vi "PrefDialog.vi"(8 "error in (no error)":errorcluster, 11 "MyPluginsBase in":refnum<class "NHRGridSim.lvclass">) -> (0 "error out":errorcluster, 1 "Save As":bool, 2 "Changed":bool, 3 "MyPluginsBase out":refnum<class "NHRGridSim.lvclass">)   [LabVIEW 2018, in "AcPwrPlugins.lvlib" / "NHRGridSim.lvclass"]
doc: "This VI opens up the modal preference dialog window and allows a user to configure the properties with new values, or keep the existing values from the last time the function was called. The user can also save the new values to a new file name and new type name using the save as button."
uses:
  NHRGridSim.lvclass
  C:/Program Files (x86)/National Instruments/LabVIEW 2018/user.lib/NIST/BaseClasses/BasePlugin_class/BasePlugin.lvclass
  C:/Users/ico/Documents/Projects/NistPluggableModules/AcPwr/AcPwrPlugins/AcPwrBaseClass/AcPwrBase.lvclass
  TypeDefs/Device(s)Settings.ctl
  TypeDefs/Modules.ctl
  Measurements.ctl
  TypeDefs/MeasurementType.ctl
  <userlib>/NIST/BaseClasses/BasePlugin_class/BasePlugin.lvclass/BasePlugin.ctl
  AcPwrBaseClass/AcPwrBase.lvclass/AcPwrBase.ctl
  <userlib>/NIST/BaseClasses/BasePlugin_class/Accessors/Read PluginIniFilePath.vi
  AcPwrBaseClass/Accessors/Read BaseConfig.vi
  AcPwrBaseClass/Accessors/Read BaseMeasurements.vi
  <userlib>/NIST/BaseClasses/BasePlugin_class/Accessors/Write PluginIniFilePath.vi
  <vilib>/Utility/config.llb/NI_LVConfig.lvlib
  AcPwrBaseClass/AcPwrBase.lvclass
panel:
  in  "Measurements":T1 {"Phase" items=["All", "A Phase", "B Phase", "C Phase"]}
  in  "Device(s)Settings":T3 {"Modules"."Phase (0: All)" items=["All", "A Phase", "B Phase", "C Phase"]; "Modules"."Mode" items=["One 3-Phase AC", "One AC", "One DC", "Three AC", "Three DC", "One 2-Phase AC and One AC", "One 2-Phase AC and One DC", "Two AC", "One AC and One DC", "Two AC and One DC", "One AC and Two DC", "One DC and One AC", "Two DC"]}
  in  "btnSaveAs":bool
  in  "Measurement RefreshTime (ms)":u32
  in  "btnSave":bool
  in  "btnCancel":bool
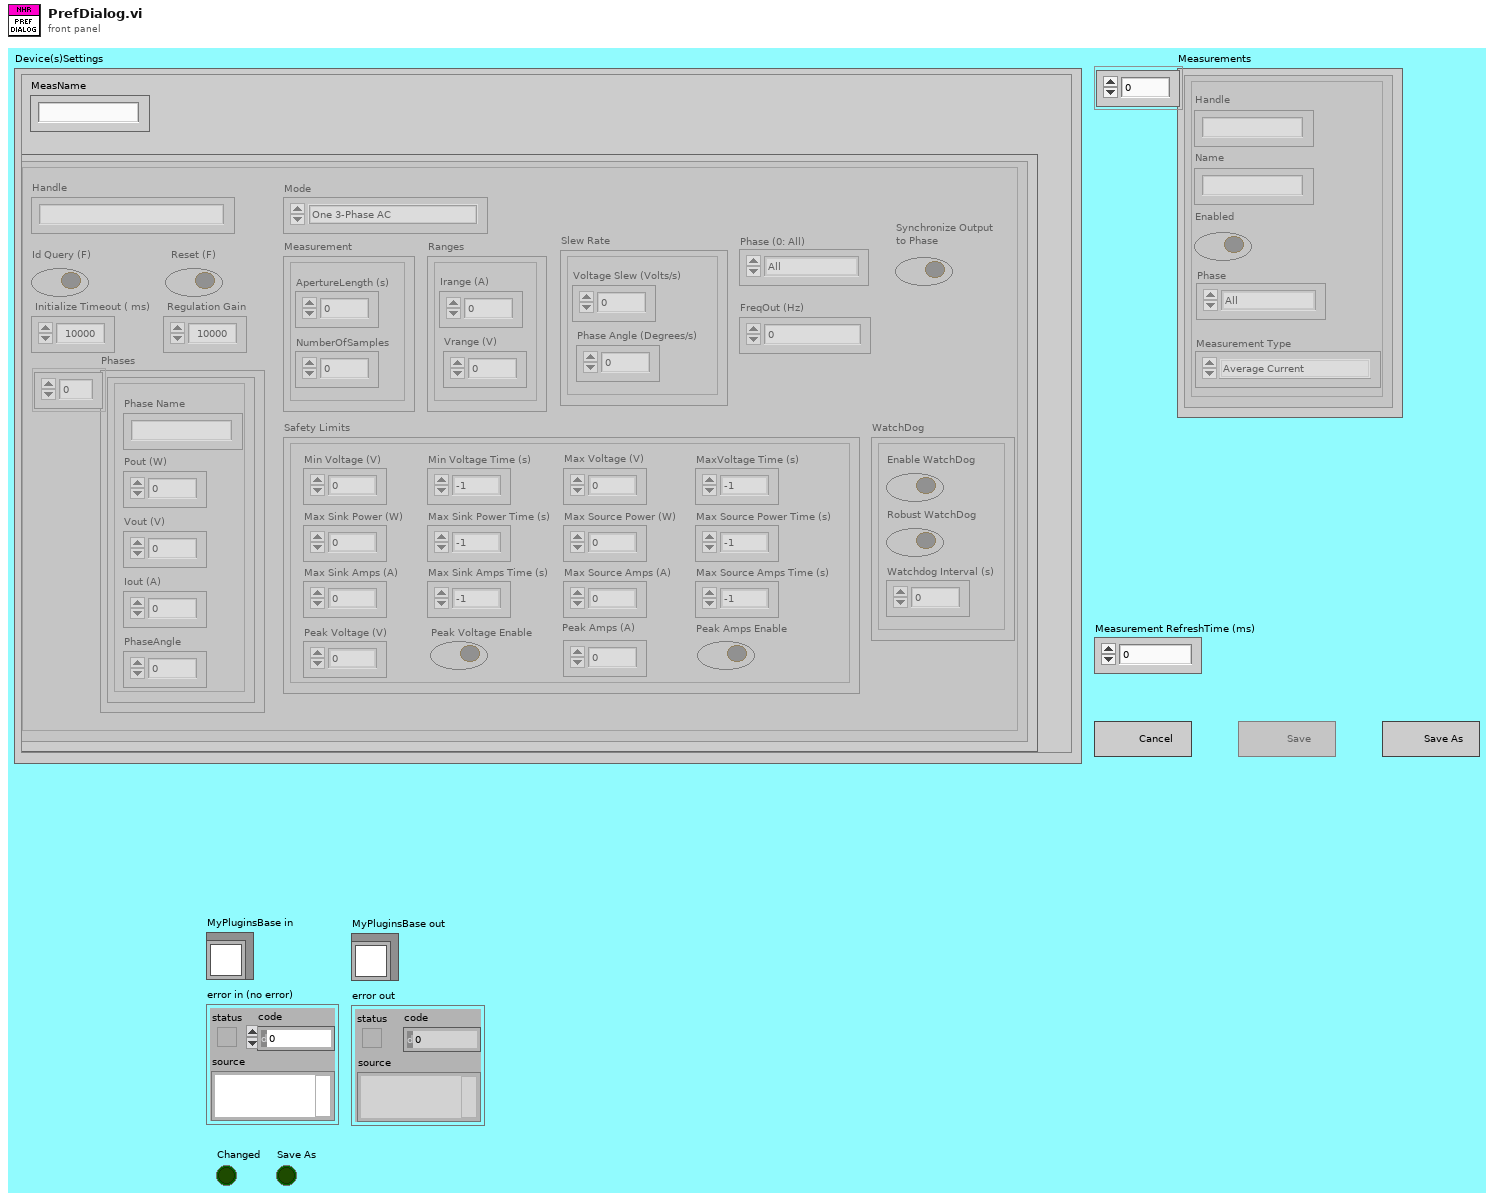
[diagram p1: front panel]
types:
  T1 = typedef "AcPwrPlugins.lvlib/NHRGridSim.lvclass/Measurements.ctl" = cluster{"Handle":string, "Name":string, "Enabled ":bool, "Measurement Value":dbl, "Phase ":i32, "Measurement Type ":T2}[]
  T2 = typedef "AcPwrPlugins.lvlib/NHRGridSim.lvclass/MeasurementType.ctl" = enum16{"Average Current", "Average Voltage"}
  T3 = typedef "AcPwrPlugins.lvlib/NHRGridSim.lvclass/Device(s)Settings.ctl" = cluster{"MeasName":string, "Modules":T4}
  T4 = typedef "AcPwrPlugins.lvlib/NHRGridSim.lvclass/Modules.ctl" = cluster{"Measurement":cluster{"ApertureLength (s)":dbl, "NumberOfSamples":u32}, "Ranges":cluster{"Irange (A)":dbl, "Vrange (V)":dbl}, "Mode":u8, "Handle":string, "FreqOut (Hz)":dbl, "Connected":bool, "btnIdQuery":bool, "btnReset":bool, "Initialize Timeout ( ms)":u32, "Phase (0: All)":i32, "WatchDog":cluster{"Enable WatchDog":bool, "Robust WatchDog":bool, "Watchdog Interval (s)":dbl}, "Safety Limits":cluster{"Min Voltage (V)":dbl, "Min Voltage Time (s)":dbl, "Max Voltage (V)":dbl, "MaxVoltage Time (s)":dbl, "Max Source Amps (A)":dbl, "Max Source Amps Time (s)":dbl, "Max Sink Amps (A)":dbl, "Max Sink Amps Time (s)":dbl, "Max Source Power (W)":dbl, "Max Source Power Time (s)":dbl, "Max Sink Power (W)":dbl, "Max Sink Power Time (s)":dbl, "Peak Voltage (V)":dbl, "Peak Voltage Enable":bool, "Peak Amps (A)":dbl, "Peak Amps Enable":bool}, "Phases":cluster{"Pout (W)":dbl, "Iout (A)":dbl, "PhaseAngle":dbl, "Vout (V)":dbl, "Phase Name":string}[], "Regulation Gain":dbl, "ChangeOntheFly":bool, "Synchronize Output \nto Phase":bool, "Slew Rate":cluster{"Voltage Slew (Volts/s)":dbl, "Phase Angle (Degrees/s)":dbl}}[]
  T5 = enum32{"Invalid", "Standard", "Closed", "Hidden", "Minimized", "Maximized"}
  T6 = enum32{"Invalid", "Default", "Floating", "Floating/Auto-Hide", "Modal"}
  T7 = enum8{"Enabled", "Disabled", "Disabled and Grayed Out"}
  T8 = typedef "AcPwrPlugins.lvlib/AcPwrBase.lvclass/BaseConfig.ctl" = cluster{"Frequency":dbl, "FrequencyRange":dbl[], "Phases":T9[], "Name":string, "PluginConfigVariant":variant, "PluginMeasVariant":variant}
  T9 = typedef "AcPwrPlugins.lvlib/AcPwrBase.lvclass/Phase.ctl" = cluster{"Name":string, "Enabled":bool, "VoltageLevel":dbl, "Handle":string, "VoltageRange":dbl[], "Connected":bool, "CurrentLimit":dbl, "Waveform":string}
  T10 = typedef "AcPwrPlugins.lvlib/AcPwrBase.lvclass/BaseMeasurements.ctl" = cluster{"Handle":string, "Name":string, "Enabled":bool, "Measurement Value":dbl, "btnMeasFetch":bool, "Chroma Hold Peak Current Measurement":bool, "Chroma Measurement Type":T11, "Chroma Protection Status String":string, "NHRDC Fetch Method":i32, "NHRDC Fetch Time (s)":sgl, "NHRDC Measurement Type":i32, "NHRGridSim Measurement Type ":enum16{"Average Current", "Max Current", "Min Current", "Average Voltage", "Max Voltage", "Min Voltage", "Average True Power", "Max True Power", "Min True Power", "Average Apparent Power", "Max Apparent Power", "Min Apparent Power", "Power Factor", "Crest Factor"}, "NHRGridSim Phase ":i32, "PPS Measurement Type ":enum16{"Voltage RMS L-N", "Voltage RMS L-L", "Frequency", "Current RMS", "Current Peak", "Crest Factor", "Power Factor", "Power VA", "Real Power"}, "PPS Channel Name":enum16{"A", "B", "C"}}[]
  T11 = typedef "AcPwrPlugins.lvlib/ChromaAcLoad.lvclass/MeasurementType.ctl" = enum16{"Voltage (Vrms or V)", "Current (Arms or A)", "Power (W)", "Peak Voltage (V)", "Peak Current (A)", "Peak Power (W)", "Frequency (Hz)", "Resistance (Ohms)", "Voltage Overshoot (V)", "Positive Peak Current (A)", "Voltage Undershoot (V)", "Negative Peak Current (A)", "Apparent Power (VA)", "Reacitive Power (VAR)", "Voltage THD", "Power Factor", "Current's Crest Factor"}
  T12 = cluster{"Measurement":cluster{"ApertureLength (s)":dbl, "NumberOfSamples":u32}, "Ranges":cluster{"Irange (A)":dbl, "Vrange (V)":dbl}, "Mode":u8, "Handle":string, "FreqOut (Hz)":dbl, "Connected":bool, "btnIdQuery":bool, "btnReset":bool, "Initialize Timeout ( ms)":u32, "Phase (0: All)":i32, "WatchDog":cluster{"Enable WatchDog":bool, "Robust WatchDog":bool, "Watchdog Interval (s)":dbl}, "Safety Limits":cluster{"Min Voltage (V)":dbl, "Min Voltage Time (s)":dbl, "Max Voltage (V)":dbl, "MaxVoltage Time (s)":dbl, "Max Source Amps (A)":dbl, "Max Source Amps Time (s)":dbl, "Max Sink Amps (A)":dbl, "Max Sink Amps Time (s)":dbl, "Max Source Power (W)":dbl, "Max Source Power Time (s)":dbl, "Max Sink Power (W)":dbl, "Max Sink Power Time (s)":dbl, "Peak Voltage (V)":dbl, "Peak Voltage Enable":bool, "Peak Amps (A)":dbl, "Peak Amps Enable":bool}, "Phases":cluster{"Pout (W)":dbl, "Iout (A)":dbl, "PhaseAngle":dbl, "Vout (V)":dbl, "Phase Name":string}[], "Regulation Gain":dbl, "ChangeOntheFly":bool, "Synchronize Output \nto Phase":bool, "Slew Rate":cluster{"Voltage Slew (Volts/s)":dbl, "Phase Angle (Degrees/s)":dbl}}
  T13 = typedef "NI_LVConfig.lvlib/Config Data RefNum.ctl" = refnum<k1>
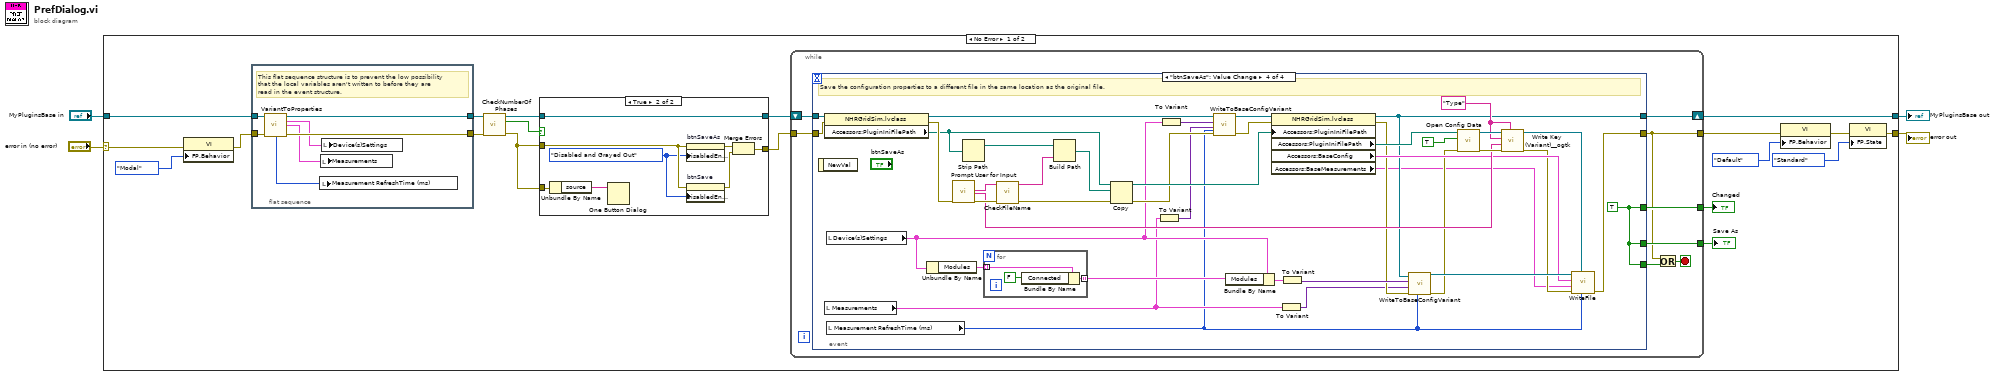
[diagram p0: block diagram]
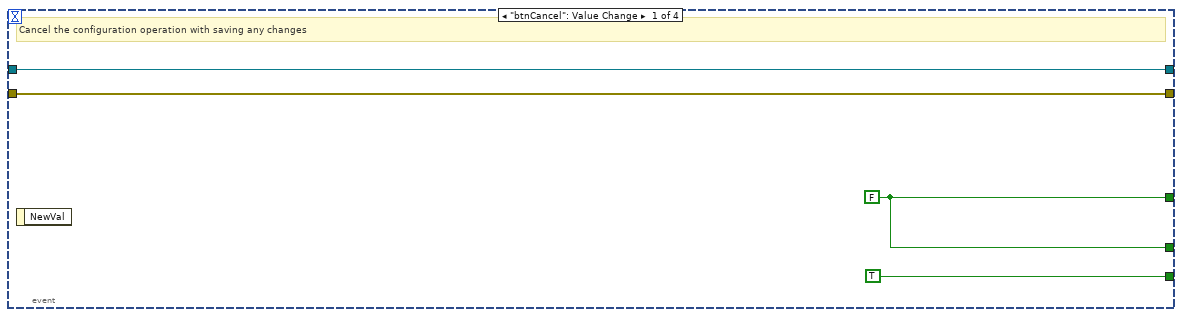
[diagram p2: hidden frame]
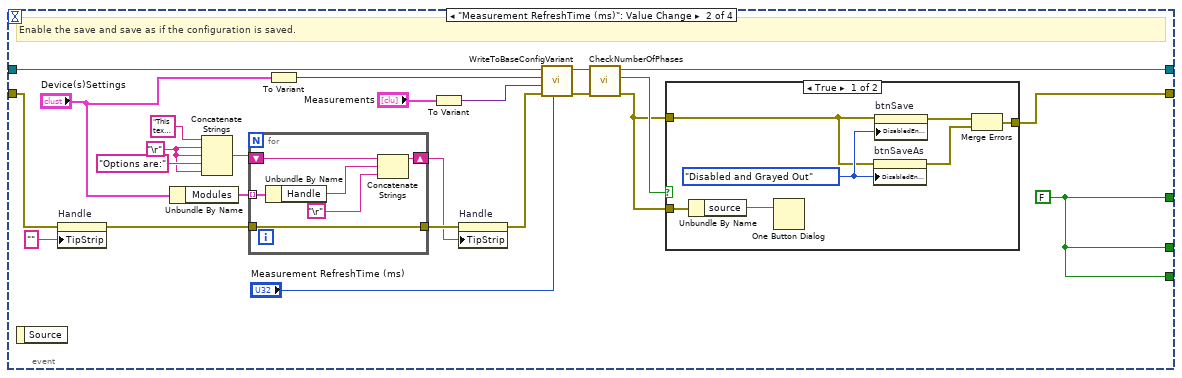
[diagram p3: hidden frame]
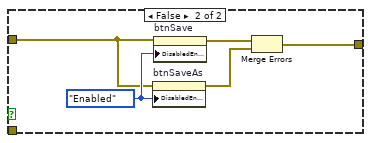
[diagram p4: hidden frame]
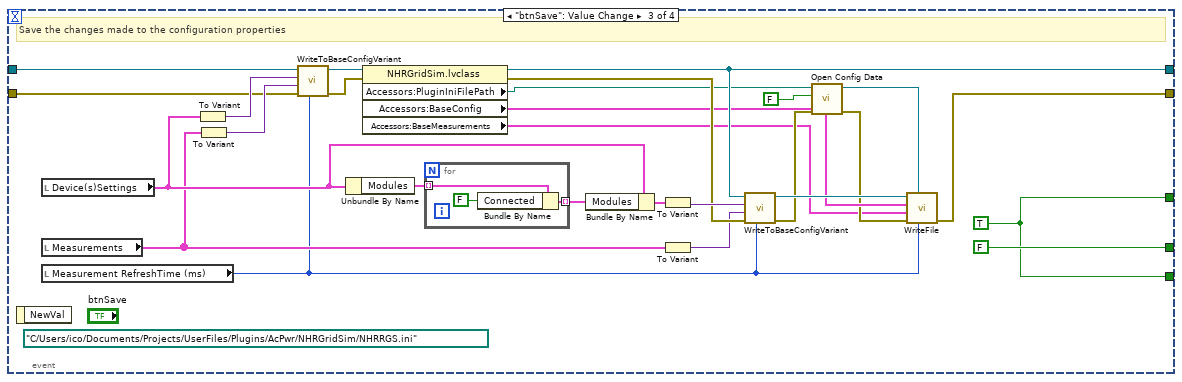
[diagram p5: hidden frame]
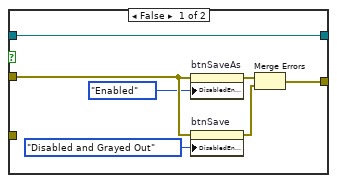
[diagram p6: hidden frame]
diagram:
  n1 = case shown="No Error" "error in (no error)" {
    selector: "error in (no error)" -> [w21 w175]
    tunnel: "MyPluginsBase in" -> [w16 w174]
    tunnel: [w14 w174] -> w2
    tunnel: [w12 w175] -> w1
    frame No Error {
      n2 = property class="VI"(error in=w21, "FP.Behavior"=T6."Modal" ("Front Panel Window:Behavior")) -> (error out=w17:errorcluster)  [unwired: 1 in, 1 out]
      n3 = flat-sequence {
        tunnel: w16 -> [w30]
        tunnel: [w29] -> w9
        tunnel: [w27] -> w10
        tunnel: w17 -> [w28]
        frame #0 {
          # "This flat sequence structure is to prevent the low possibility that the local variables aren't written to before they are read in the event structure."
          n4 = call "VariantToProperties.vi"("NHRGridSim in"=w30, "error in (no error)"=w28) -> ("NHRGridSim out"=w29:refnum<class "NHRGridSim.lvclass">, "Device(s)Settings"=w26:T3, "Measurements"=w24:T1, "Measurement Refresh Time (ms)"=w25:u32, "error out"=w27:errorcluster)  [unwired: 7 in, 2 out]
          n5 = local write "Measurement RefreshTime (ms)"(w25) -> ()
          n6 = local write "Measurements"(w24) -> ()
          n7 = local write "Device(s)Settings"(w26) -> ()
        }
      }
      n8 = call "CheckNumberOfPhases.vi"("error in (no error)"=w10, "NHRGridSim in"=w9) -> ("error out"=w7:errorcluster, "Boolean"=w8:bool, "NHRGridSim out"=w6:refnum<class "NHRGridSim.lvclass">)  [unwired: 6 in, 1 out]
      n9 = case shown="True" w8 {
        tunnel: w7 -> [w164 w172]
        tunnel: [w163 w171] -> w15
        tunnel: w7 -> [_ w168]
        tunnel: w6 -> [w159 w166]
        tunnel: [w159 w166] -> w5
        frame False {
          # "Check if the number of Phases=Loads. If no disables the ability\nto save as."
          n10 = property on="btnSaveAs" class="Bool"(error in=w164, "DisabledEnum"=T7."Enabled" ("Disabled")) -> (error out=w165:errorcluster)  [unwired: 1 in, 1 out]
          n11 = property on="btnSave" class="Bool"(error in=w164, "DisabledEnum"=T7."Disabled and Grayed Out" ("Disabled")) -> (error out=w162:errorcluster)  [unwired: 1 in, 1 out]
          n12 = Merge Errors(w165, w162) -> (w163:errorcluster)
        }
        frame True {
          w169 = T7."Disabled and Grayed Out" ("Disabled")
          # "Check if the number of Phases=Loads. If no disables the ability\nto save as."
          n13 = Unbundle By Name(w168) -> ("source"=w167:string)
          n14 = One Button Dialog(message=w167) -> ()  [unwired: 1 in, 1 out]
          n15 = property on="btnSaveAs" class="Bool"(error in=w172, "DisabledEnum"=w169) -> (error out=w173:errorcluster)  [unwired: 1 in, 1 out]
          n16 = property on="btnSave" class="Bool"(error in=w172, "DisabledEnum"=w169) -> (error out=w170:errorcluster)  [unwired: 1 in, 1 out]
          n17 = Merge Errors(w173, w170) -> (w171:errorcluster)
        }
      }
      n18 = while {
        shift-right: [w36] -> w14
        shift-left: w5 -> [w37]
        tunnel: [w38] -> w22
        tunnel: [w34] -> w13
        tunnel: w15 -> [w35]
        tunnel: [w31] -> w11
        stop <- w33 stop-if-true
        n19 = event shown="[3] \"btnSaveAs\": Value Change" {
          selector: _ -> [_ _ _ _]
          dyn-events: _ -> [_ _ _ _]
          timeout: _ -> [_ _ _ _]
          tunnel: [w39 w65 w109 w150] -> w38
          tunnel: [TRUE w65 w109 w150] -> w32
          tunnel: w37 -> [w41 w57 w90 w144]
          tunnel: [w41 w60 w104 w128] -> w36
          tunnel: [w40 w66 w106 w130] -> w31
          tunnel: w35 -> [w40 w50 w87 w143]
          tunnel: [w39 w65 FALSE w150] -> w34
          event "btnCancel": Value Change {
            w39 = FALSE
            # "Cancel the configuration operation with saving any changes"
            n20 = event-data() -> ()  [unwired: 1 in, 1 out]
          }
          event "Measurement RefreshTime (ms)": Value Change {
            w62 = "\r"
            w65 = FALSE
            # "Enable the save and save as if the configuration is saved."
            n21 = event-data() -> ()  [unwired: 1 in, 1 out]
            n22 = property on="Handle" class="Str"(error in=w50, "TipStrip"="" ("Tip Strip")) -> (error out=w49:errorcluster)  [unwired: 1 in, 1 out]
            n23 = Unbundle By Name("Device(s)Settings") -> ("Modules"=w53:T4)
            n24 = Concatenate Strings("This text in this handle of the instrument and entered in the  \nhandle control in the Phases array EXACTLY, lest the attempt \nto interact with the instrument will fail.", w62, w62, "Options are:" ("Handle"), w62) -> (w61:string)
            n25 = for {
              shift-right: [w72] -> w46
              shift-left: w61 -> [w71]
              tunnel: w53 -> [w70] mode=indexing
              tunnel: w49 -> [w67]
              tunnel: [w67] -> w47
              n26 = Unbundle By Name(w70) -> ("Handle"=w69:string)
              n27 = Concatenate Strings(w71, w69, "\r") -> (w72:string)
            }
            n28 = To Variant(anything="Device(s)Settings") -> (Variant=w58:variant)
            n29 = To Variant(anything="Measurements") -> (Variant=w43:variant)
            n30 = property on="Handle" class="Str"(error in=w47, "TipStrip"=w46) -> (error out=w48:errorcluster)  [unwired: 1 in, 1 out]
            n31 = call "WriteToBaseConfigVariant.vi"("Measurement RefreshTime (ms)"="Measurement RefreshTime (ms)", "error in (no error)"=w48, "Meas"=w43, "Config"=w58, "NHRGridSim in"=w57) -> ("error out"=w55:errorcluster, "NHRGridSim out"=w56:refnum<class "NHRGridSim.lvclass">)  [unwired: 5 in]
            n32 = call "CheckNumberOfPhases.vi"("error in (no error)"=w55, "NHRGridSim in"=w56) -> ("error out"=w54:errorcluster, "Boolean"=w59:bool, "NHRGridSim out"=w60:refnum<class "NHRGridSim.lvclass">)  [unwired: 6 in, 1 out]
            n33 = case shown="True" w59 {
              tunnel: w54 -> [w76 w81]
              tunnel: [w75 w80] -> w66
              tunnel: w54 -> [w73 _]
              frame True {
                w77 = T7."Disabled and Grayed Out" ("Disabled")
                n34 = Unbundle By Name(w73) -> ("source"=w74:string)
                n35 = One Button Dialog(message=w74) -> ()  [unwired: 1 in, 1 out]
                n36 = property on="btnSaveAs" class="Bool"(error in=w76, "DisabledEnum"=w77) -> (error out=w79:errorcluster)  [unwired: 1 in, 1 out]
                n37 = property on="btnSave" class="Bool"(error in=w76, "DisabledEnum"=w77) -> (error out=w78:errorcluster)  [unwired: 1 in, 1 out]
                n38 = Merge Errors(w78, w79) -> (w75:errorcluster)
              }
              frame False {
                w82 = T7."Enabled" ("Disabled")
                n39 = property on="btnSaveAs" class="Bool"(error in=w81, "DisabledEnum"=w82) -> (error out=w84:errorcluster)  [unwired: 1 in, 1 out]
                n40 = property on="btnSave" class="Bool"(error in=w81, "DisabledEnum"=w82) -> (error out=w83:errorcluster)  [unwired: 1 in, 1 out]
                n41 = Merge Errors(w83, w84) -> (w80:errorcluster)
              }
            }
          }
          event "btnSave": Value Change {
            (unwired) path "C:/Users/ico/Documents/Projects/UserFiles/Plugins/AcPwr/NHRGridSim/NHRRGS.ini" ("Accessors:PluginIniFilePath")
            w109 = TRUE ("StartMeas")
            # "Save the changes made to the configuration properties"
            n42 = event-data() -> ()  [unwired: 1 in, 1 out]
            n43 = local read "Device(s)Settings"() -> (w89:T3)
            n44 = local read "Measurements"() -> (w88:T1)
            n45 = local read "Measurement RefreshTime (ms)"() -> (w86:u32)
            n46 = To Variant(anything=w89) -> (Variant=w94:variant)
            n47 = To Variant(anything=w88) -> (Variant=w93:variant)
            n48 = call "WriteToBaseConfigVariant.vi"("Measurement RefreshTime (ms)"=w86, "error in (no error)"=w87, "Meas"=w93, "Config"=w94, "NHRGridSim in"=w90) -> ("error out"=w91:errorcluster, "NHRGridSim out"=w92:refnum<class "NHRGridSim.lvclass">)  [unwired: 5 in]
            n49 = Unbundle By Name(w89) -> ("Modules"=w107:T4)
            n50 = property class="NHRGridSim.lvclass"(reference=w92, error in=w91) -> (reference out=w104:refnum<class "NHRGridSim.lvclass">, error out=w101:errorcluster, "Accessors:PluginIniFilePath"=w85:path, "Accessors:BaseConfig"=w100:T8, "Accessors:BaseMeasurements"=w97:T10)
            n51 = for {
              tunnel: w107 -> [w114] mode=indexing
              tunnel: [w113] -> w108 mode=indexing
              n52 = Bundle By Name(cluster=w114, "Connected"=FALSE) -> (w113:T12)
            }
            n53 = Bundle By Name(cluster=w89, "Modules"=w108) -> (w96:T3)
            n54 = To Variant(anything=w96) -> (Variant=w105:variant)
            n55 = To Variant(anything=w88) -> (Variant=w95:variant)
            n56 = call "WriteToBaseConfigVariant.vi"("Measurement RefreshTime (ms)"=w86, "error in (no error)"=w101, "Meas"=w95, "Config"=w105, "NHRGridSim in"=w104) -> ("error out"=w102:errorcluster, "NHRGridSim out"=w103:refnum<class "NHRGridSim.lvclass">)  [unwired: 5 in]
            n57 = call <vilib>:"Open Config Data.vi"("error in (no error)"=w102, "create file if necessary (T)"=FALSE, "configuration file path"=w85) -> ("error out"=w98:errorcluster, "refnum"=w99:T13)  [unwired: 6 in, 1 out]
            n58 = call-dynamic "WriteFile.vi"("RefreshTime"=w86, "Refnum in"=w99, "error in (no error)"=w98, "BaseMeasurements"=w97, "BaseConfiguration"=w100, "NHRGridSim in"=w103) -> ("error out"=w106:errorcluster)  [unwired: 4 in, 1 out]
          }
          event "btnSaveAs": Value Change {
            w145 = "Type" ("section (optional)")
            w150 = TRUE
            # "Save the configuration properties to a different file in the same location as the original file."
            n59 = event-data() -> ()  [unwired: 1 in, 1 out]
            n60 = property class="NHRGridSim.lvclass"(reference=w144, error in=w143) -> (reference out=w120:refnum<class "NHRGridSim.lvclass">, error out=w142:errorcluster, "Accessors:PluginIniFilePath"=w141:path)
            n61 = local read "Measurements"() -> (w117:T1)
            n62 = local read "Device(s)Settings"() -> (w118:T3)
            n63 = local read "Measurement RefreshTime (ms)"() -> (w115:u32)
            n64 = Unbundle By Name(w118) -> ("Modules"=w138:T4)
            n65 = call "Prompt User for Input"("error in (no error)"=w142) -> ("File Name"=w140:string, "PluginType"=w146:string, "error out"=w147:errorcluster)  [unwired: 15 in, 1 out]
            n66 = Strip Path(path=w141) -> (stripped path=w152:path)  [unwired: 1 out]
            n67 = for {
              tunnel: w138 -> [w158] mode=indexing
              tunnel: [w157] -> w139 mode=indexing
              n68 = Bundle By Name(cluster=w158, "Connected"=FALSE) -> (w157:T12)
            }
            n69 = call "CheckFileName.vi"("Error In"=w147, "File Name in"=w140) -> ("Error Out"=w148:errorcluster, "File Name out"=w149:string)  [unwired: 8 in]
            n70 = Build Path(base path=w152, name or relative path=w149) -> (appended path=w151:path)
            n71 = Copy(8:w148, 10:w151, 11:w141) -> (0:w123:errorcluster, 3:w134:path)  [unwired: 2 in, 1 out]
            n72 = To Variant(anything=w117) -> (Variant=w116:variant)
            n73 = To Variant(anything=w118) -> (Variant=w119:variant)
            n74 = call "WriteToBaseConfigVariant.vi"("Measurement RefreshTime (ms)"=w115, "error in (no error)"=w123, "Meas"=w116, "Config"=w119, "NHRGridSim in"=w120) -> ("error out"=w122:errorcluster, "NHRGridSim out"=w121:refnum<class "NHRGridSim.lvclass">)  [unwired: 5 in]
            n75 = Bundle By Name(cluster=w118, "Modules"=w139) -> (w137:T3)
            n76 = property class="NHRGridSim.lvclass"(reference=w121, error in=w122, "Accessors:PluginIniFilePath"=w134) -> (reference out=w128:refnum<class "NHRGridSim.lvclass">, error out=w129:errorcluster, "Accessors:PluginIniFilePath"=w133:path, "Accessors:BaseConfig"=w132:T8, "Accessors:BaseMeasurements"=w125:T10)
            n77 = To Variant(anything=w117) -> (Variant=w124:variant)
            n78 = To Variant(anything=w137) -> (Variant=w136:variant)
            n79 = call "WriteToBaseConfigVariant.vi"("Measurement RefreshTime (ms)"=w115, "error in (no error)"=w129, "Meas"=w124, "Config"=w136, "NHRGridSim in"=w128) -> ("error out"=w127:errorcluster, "NHRGridSim out"=w135:refnum<class "NHRGridSim.lvclass">)  [unwired: 5 in]
            n80 = call <vilib>:"Open Config Data.vi"("error in (no error)"=w127, "create file if necessary (T)"=TRUE, "configuration file path"=w133) -> ("error out"=w154:errorcluster, "refnum"=w153:T13)  [unwired: 6 in, 1 out]
            n81 = call <userlib>:"Write Key (Variant)__ogtk.vi"("section"=w145, "error in (no error)"=w154, "key-value"=w146, "key (optional)"=w145, "refnum"=w153) -> ("error out"=w126:errorcluster, "refnum out"=w131:T13)  [unwired: 5 in]
            n82 = call-dynamic "WriteFile.vi"("RefreshTime"=w115, "Refnum in"=w131, "error in (no error)"=w126, "BaseMeasurements"=w125, "BaseConfiguration"=w132, "NHRGridSim in"=w135) -> ("error out"=w130:errorcluster)  [unwired: 4 in, 1 out]
          }
        }
        n83 = Or(x=w31, y=w32) -> (x .or. y?=w33:bool)
      }
      "Changed" <- w22
      "Save As" <- w13
      n84 = property class="VI"(error in=w11, "FP.Behavior"=T6."Default" ("Front Panel Window:Behavior")) -> (error out=w20:errorcluster)  [unwired: 1 in, 1 out]
      n85 = property class="VI"(error in=w20, "FP.State"=T5."Standard" ("Front Panel Window:State")) -> (error out=w12:errorcluster)  [unwired: 1 in, 1 out]
    }
    frame Error {
    }
  }
  "MyPluginsBase out" <- w2
  "error out" <- w1
